vi "Configure Export Signal.vi"(8 "error in (no error)":errorcluster, 11 "object in":refnum<class "Fetch Waveforms CFG.lvclass">) -> (0 "error out":errorcluster, 3 "object out":refnum<class "Fetch Waveforms CFG.lvclass">)   [LabVIEW 2023, in "Scope Simulated CFGs.lvlib" / "Fetch Waveforms CFG.lvclass"]
uses:
  Fetch Waveforms CFG.lvclass
  D:/git/HAL/HAL GOOP4/Configuration JSON Base/CFG JSON Base.lvclass
  <instrlib>/niScope/Controls/niScope export destinations.ctl
  42599f19-f05a-4c63-9b72-d5b944f4c65f.vi
  <vilib>/JDP Science/JSONtext/Find Item.vi
  <vilib>/JDP Science/JSONtext/Next JSON Value.vi
  <vilib>/JDP Science/JSONtext/String Subset.vi
  <vilib>/JDP Science/JSONtext/Parsing/Advance past next JSON Value (inlined COPY).vi
  <vilib>/JDP Science/JSONtext/Parsing/Advance past whitespace.vi
  <vilib>/JDP Science/JSONtext/Parsing/Advance past String.vi
  <vilib>/JDP Science/JSONtext/Parsing/Advance past Number.vi
  <vilib>/JDP Science/JSONtext/Parsing/Advance past Line Ending.vi
  <vilib>/JDP Science/JSONtext/Parsing/Parse Full Path or Item Name.vi
  <vilib>/JDP Science/JSONtext/Parsing/Advance past Array.vi
  <vilib>/JDP Science/JSONtext/Parsing/Advance past Object.vi
  <vilib>/JDP Science/JSONtext/support/Error Cluster From Code.vi
  <vilib>/JDP Science/JSONtext/Offset/Find Item Locations by Path.vi
  <vilib>/JDP Science/JSONtext/JSON text to Variant.vi
  <vilib>/Utility/error.llb/Error Cluster From Error Code.vi
  <vilib>/JDP Science/JSONtext/LVClass Serializer/JSONtext LVClass Serializer.lvclass
  <vilib>/ErrorRing/Error Ring.xnode
  Configuration JSON Base/CFG JSON Base.lvclass
panel:
  out "Data":T2
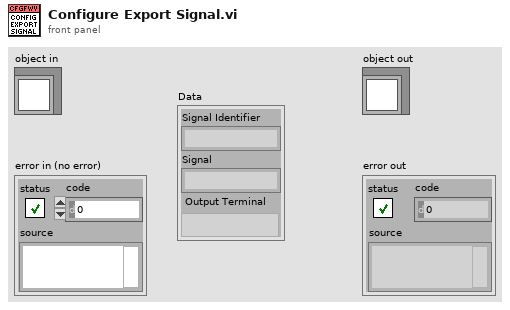
[diagram p1: front panel]
types:
  T1 = typedef "niScope export destinations.ctl" = string
  T2 = cluster{"Signal Identifier":string, "Signal":string, "Output Terminal":T1}
  T3 = cluster{"Signal Identifier":string, "Signal":string, "Output Terminal":string}
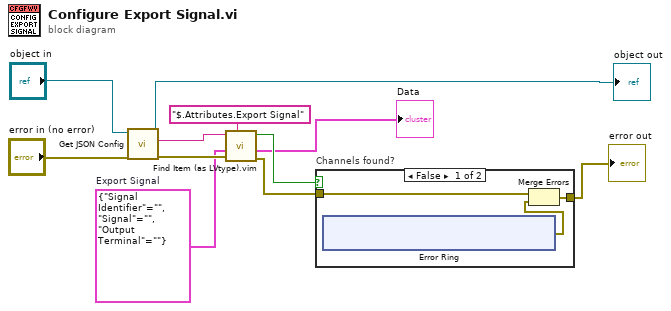
[diagram p0: block diagram]
diagram:
  w7 = T3 {"Signal Identifier"="", "Signal"="", "Output Terminal"=""}  # Export Signal
  n1 = call "Get JSON Config.vi"("error in (no error)"="error in (no error)", "CFG Base in"="object in") -> ("error out"=w10:errorcluster, "<JSON>Config>"=w9:string, "CFG Base out"=→"object out":refnum<class "Fetch Waveforms CFG.lvclass">)  [unwired: 7 in]
  n2 = call "Find Item (as LVtype).vim"("$Path or Item Name"="$.Attributes.Export Signal", "error in (no error)"=w10, "Data Type and Default Value"=w7, "JSON"=w9) -> ("error out"=w6:errorcluster, "Data"=→"Data":T3, "Found"=w5:bool)  [unwired: 4 in, 1 out]
  n3 = case "Channels found?" shown="False" w5 {
    tunnel: [w14 w20] -> w2
    tunnel: w6 -> [w12 w20]
    frame False {
      n4 = xnode "Error Ring"() -> ("error out"=w13:errorcluster)
      n5 = Merge Errors(w12, w13) -> (w14:errorcluster)
    }
    frame True {
    }
  }
  "error out" <- w2
